vi "tvac_gui_test.vi"() -> ()   [LabVIEW 2017]
panel:
  in  "Tab Control":enum32{"Page 1", "Page 2"}(tab)
  out "Cluster":T1
  out "XY Graph":cluster{"X":dbl, "Y":dbl}[](graph)
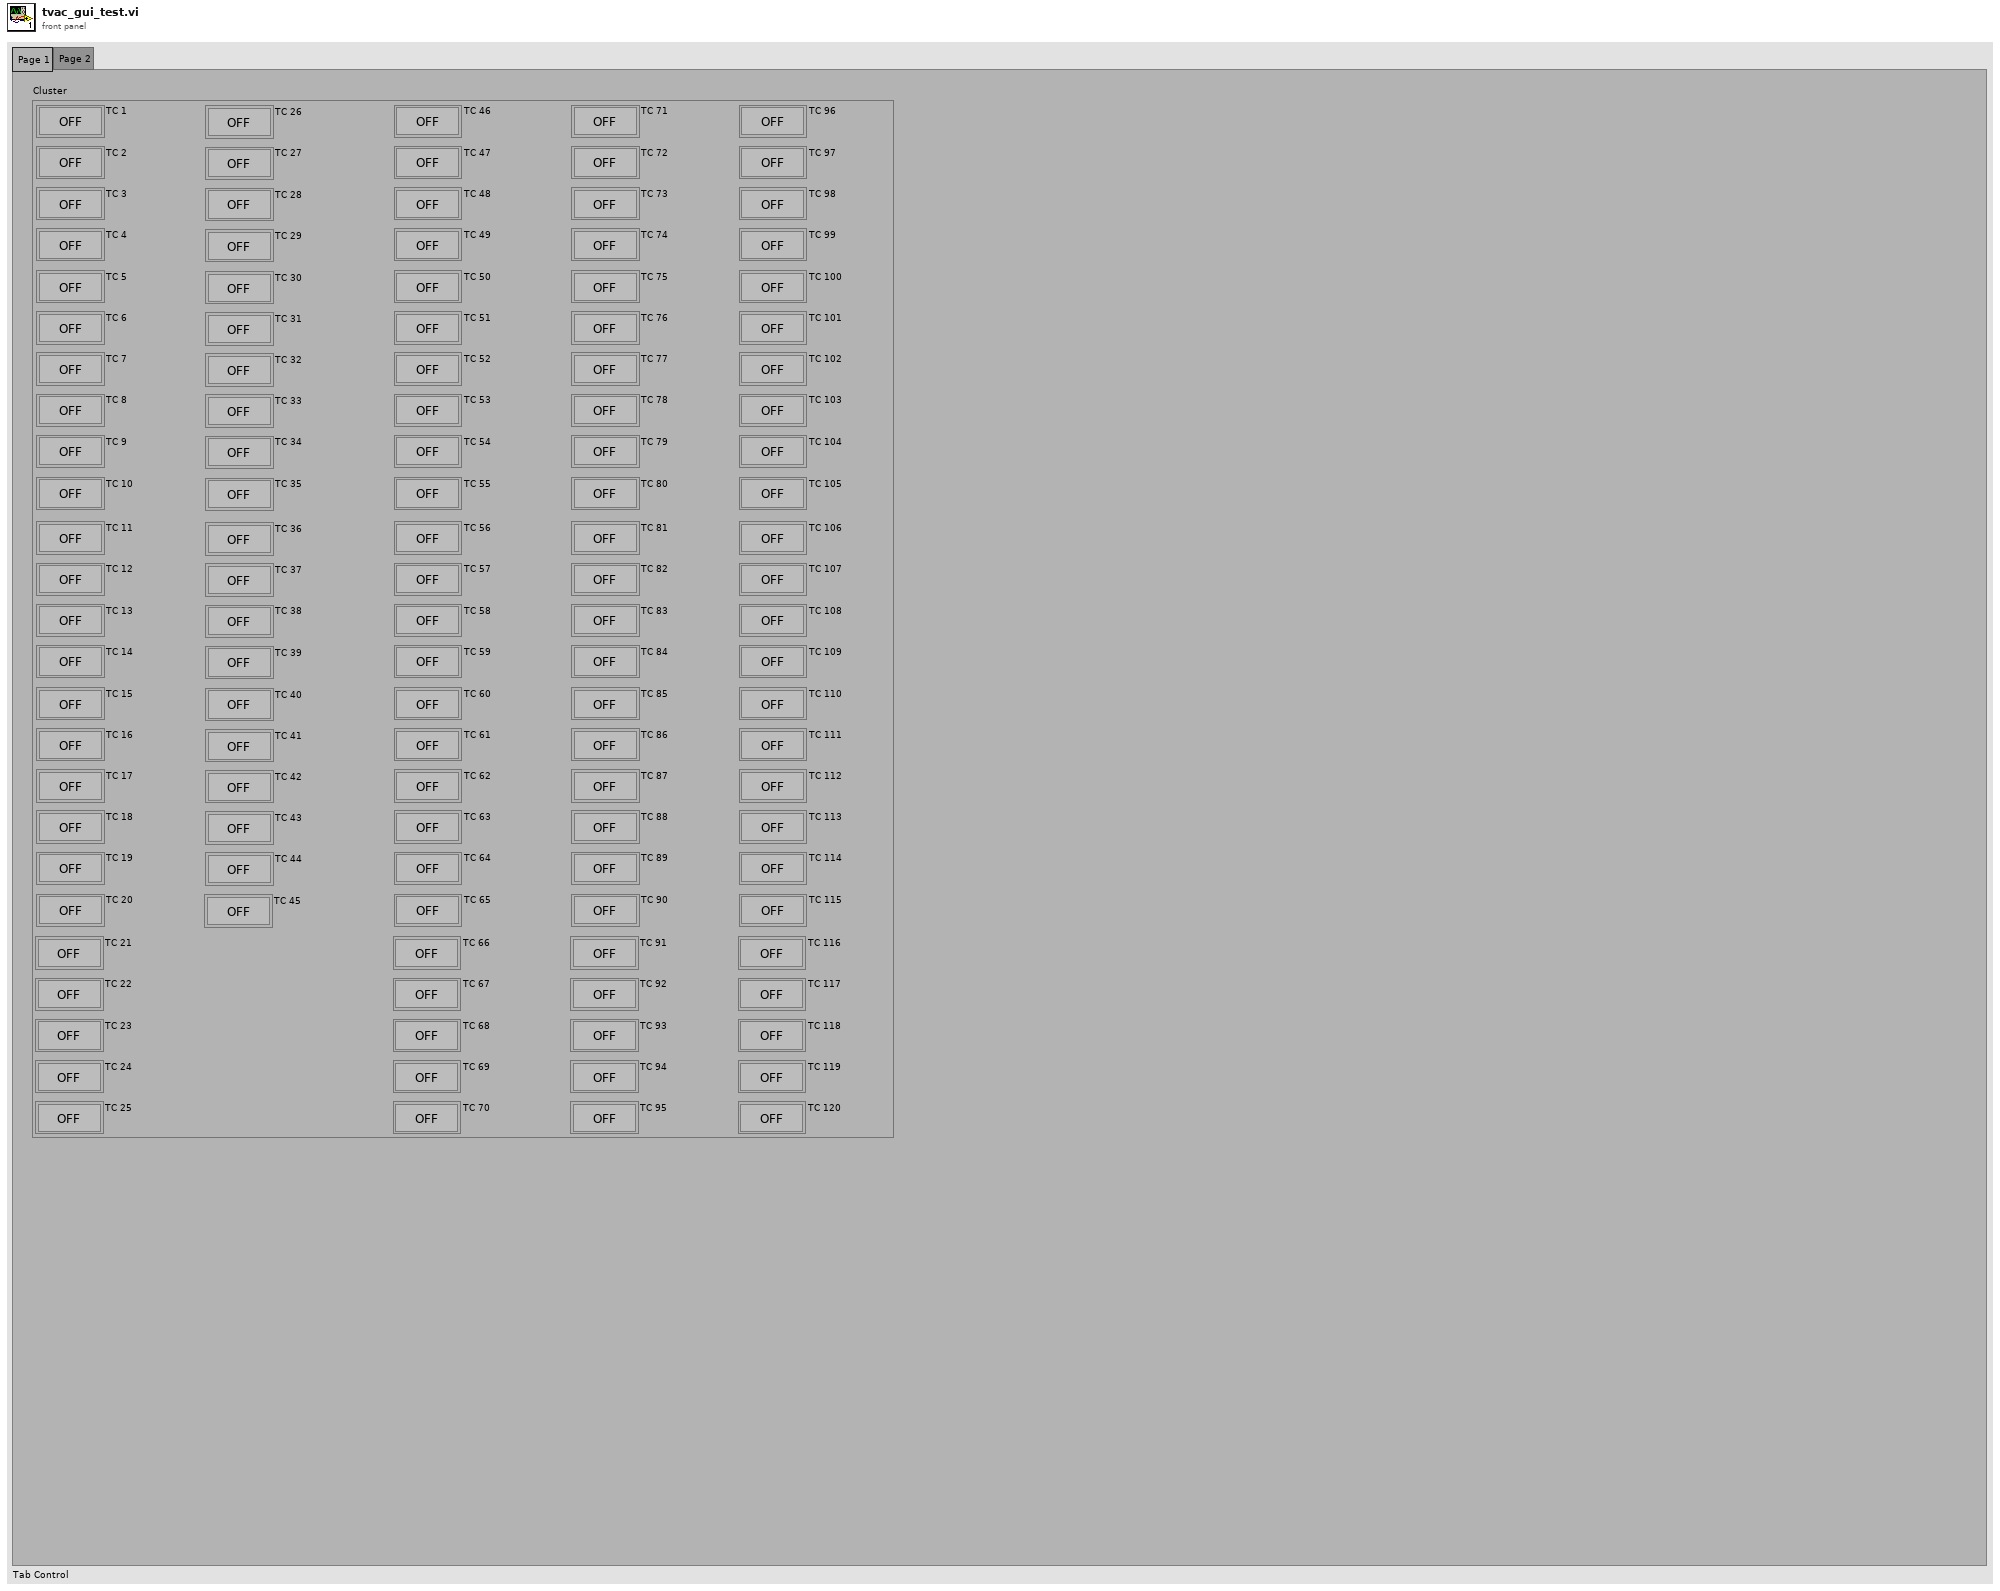
[diagram p1: front panel]
types:
  T1 = cluster{"TC 1":bool, "TC 2":bool, "TC 3":bool, "TC 4":bool, "TC 5":bool, "TC 6":bool, "TC 7":bool, "TC 8":bool, "TC 9":bool, "TC 10":bool, "TC 11":bool, "TC 12":bool, "TC 13":bool, "TC 14":bool, "TC 15":bool, "TC 16":bool, "TC 17":bool, "TC 18":bool, "TC 19":bool, "TC 20":bool, "TC 21":bool, "TC 22":bool, "TC 23":bool, "TC 24":bool, "TC 25":bool, "TC 26":bool, "TC 27":bool, "TC 28":bool, "TC 29":bool, "TC 30":bool, "TC 31":bool, "TC 32":bool, "TC 33":bool, "TC 34":bool, "TC 35":bool, "TC 36":bool, "TC 37":bool, "TC 38":bool, "TC 39":bool, "TC 40":bool, "TC 41":bool, "TC 42":bool, "TC 43":bool, "TC 44":bool, "TC 45":bool, "TC 46":bool, "TC 47":bool, "TC 48":bool, "TC 49":bool, "TC 50":bool, "TC 51":bool, "TC 52":bool, "TC 53":bool, "TC 54":bool, "TC 55":bool, "TC 56":bool, "TC 57":bool, "TC 58":bool, "TC 59":bool, "TC 60":bool, "TC 61":bool, "TC 62":bool, "TC 63":bool, "TC 64":bool, "TC 65":bool, "TC 66":bool, "TC 67":bool, "TC 68":bool, "TC 69":bool, "TC 70":bool, "TC 71":bool, "TC 72":bool, "TC 73":bool, "TC 74":bool, "TC 75":bool, "TC 76":bool, "TC 77":bool, "TC 78":bool, "TC 79":bool, "TC 80":bool, "TC 81":bool, "TC 82":bool, "TC 83":bool, "TC 84":bool, "TC 85":bool, "TC 86":bool, "TC 87":bool, "TC 88":bool, "TC 89":bool, "TC 90":bool, "TC 91":bool, "TC 92":bool, "TC 93":bool, "TC 94":bool, "TC 95":bool, "TC 96":bool, "TC 97":bool, "TC 98":bool, "TC 99":bool, "TC 100":bool, "TC 101":bool, "TC 102":bool, "TC 103":bool, "TC 104":bool, "TC 105":bool, "TC 106":bool, "TC 107":bool, "TC 108":bool, "TC 109":bool, "TC 110":bool, "TC 111":bool, "TC 112":bool, "TC 113":bool, "TC 114":bool, "TC 115":bool, "TC 116":bool, "TC 117":bool, "TC 118":bool, "TC 119":bool, "TC 120":bool}
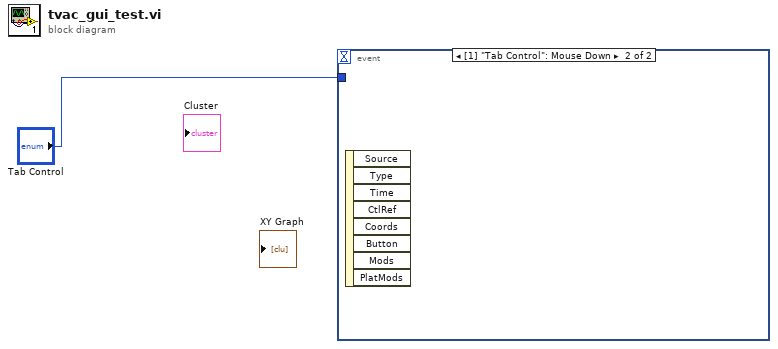
[diagram p0: block diagram]
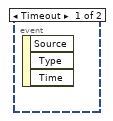
[diagram p2: hidden frame]
diagram:
  n1 = event shown="[1] \"Tab Control\": Mouse Down" {
    selector: _ -> [_ _]
    dyn-events: _ -> [_ _]
    timeout: _ -> [_ _]
    tunnel: "Tab Control" -> [_ _]
    event Timeout {
      n2 = event-data() -> ()  [unwired: 1 in, 3 out]
    }
    event "Tab Control": Mouse Down {
      n3 = event-data() -> ()  [unwired: 1 in, 8 out]
    }
  }
